vi "Script Work VIs.vi"(6 "Context":refnum<vi>, 7 "New Block Config":T1={"Name"="", "Actions"={"Init"=FALSE, "Start"=FALSE, "Run"=TRUE, "Stop"=FALSE, "Close"=FALSE}, "IO Control"=FALSE, "New Project?"=FALSE, "Project"=refnum}, 8 "error in (no error)":errorcluster, 11 "Worker Library Path":path) -> (0 "error out":errorcluster)   [LabVIEW 2022 SP3, in "FlexBlocks Support.lvlib"]
uses:
  FlexBlocks Support.lvlib
  <vilib>/Utility/traverseref.llb/TRef TravTarget.ctl
  Worker Action.ctl
  <vilib>/Utility/error.llb/Trim Whitespace One-Sided.vi
  <vilib>/Utility/traverseref.llb/VI Scripting - Traverse.lvlib
  Action Selections.ctl
  New Block Config.ctl
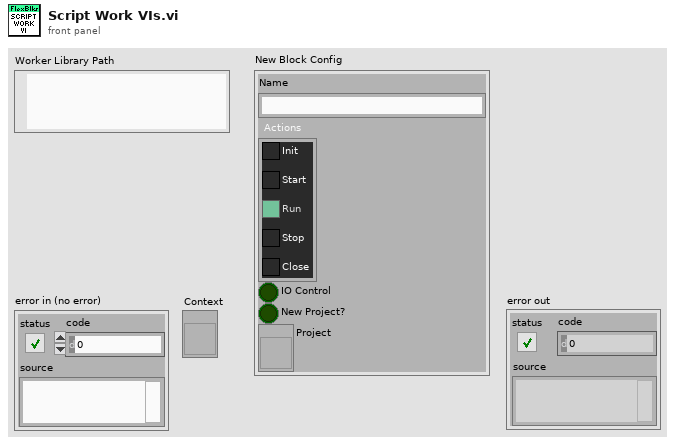
[diagram p1: front panel]
types:
  T1 = typedef "FlexBlocks Support.lvlib/New Block Config.ctl" = cluster{"Name":string, "Actions":T2, "IO Control":bool, "New Project?":bool, "Project":refnum<vi>}
  T2 = typedef "FlexBlocks Support.lvlib/Action Selections.ctl" = cluster{"Init":bool, "Start":bool, "Run":bool, "Stop":bool, "Close":bool}
  T3 = enum32{"invalid lock state", "Not Locked", "Locked (No Password)", "Password-protected"}
  T4 = typedef "TRef TravTarget.ctl" = enum16{"FP", "BD", "Other"}
  T5 = typedef "FlexBlocks Support.lvlib/Worker Action.ctl" = enum16{"Init", "Start", "Run", "Stop", "Close"}
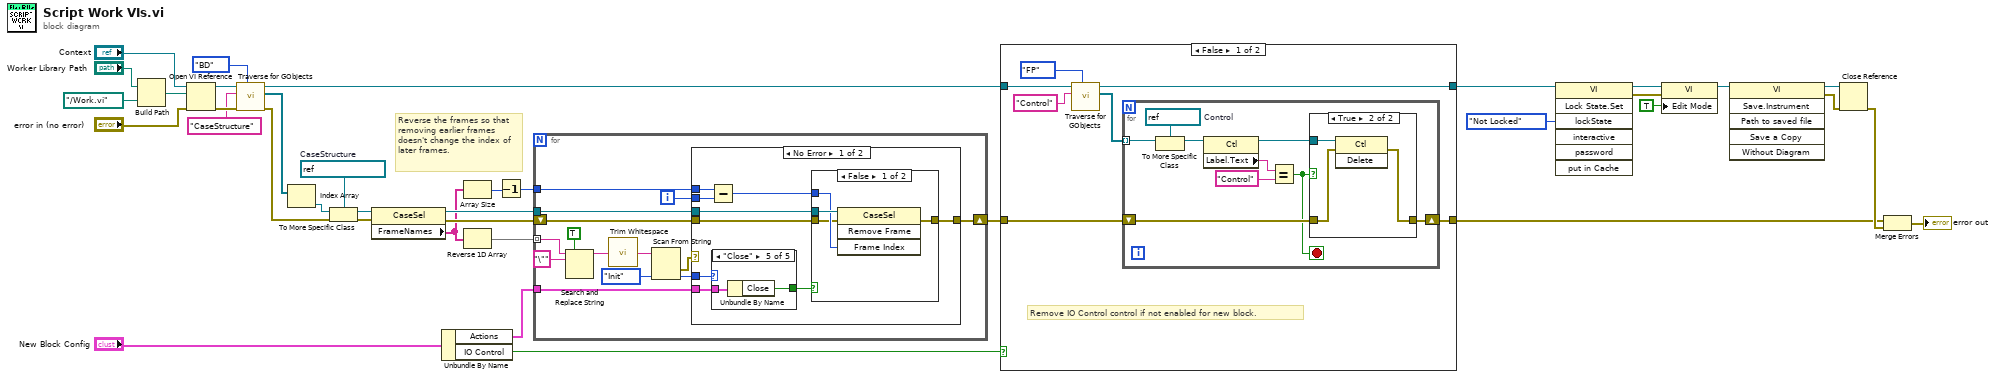
[diagram p0: block diagram]
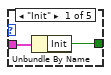
[diagram p5: hidden frame]
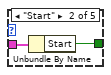
[diagram p6: hidden frame]
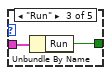
[diagram p7: hidden frame]
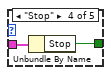
[diagram p8: hidden frame]
diagram:
  w27 = refnum<vi> refnum  # CaseStructure
  # "Reverse the frames so that removing earlier frames doesn't change the index of later frames."
  n1 = Build Path(base path="Worker Library Path", name or relative path=path "../Work.vi") -> (appended path=w35:path)
  n2 = Open VI Reference(application reference (local)="Context", vi path=w35, error in (no error)="error in (no error)") -> (vi reference=w33:refnum<vi>, error out=w31:errorcluster)  [unwired: 3 in]
  n3 = call <vilib>:"Traverse for GObjects.vi"("Traverse Target"=TRef_TravTarget."BD", "error in (no error)"=w31, "Class Name"="CaseStructure", "VI Refnum"=w33) -> ("error out"=w25:errorcluster, "References"=w29:refnum<vi>[], "dup VI Refnum"=w4:refnum<vi>)  [unwired: 4 in, 1 out]
  n4 = Index Array(array=w29) -> (element=w28:refnum<vi>)  [unwired: 1 in]
  n5 = To More Specific Class(target class=w27, reference=w28, error in=w25) -> (specific class reference=w26:refnum<vi>, error out=w24:errorcluster)
  n6 = property class="CaseSel"(reference=w26, error in=w24) -> (reference out=w23:refnum<vi>, error out=w22:errorcluster, "FrameNames"=w15:string[])
  n7 = Unbundle By Name("New Block Config") -> ("Actions"=w6:T2, "IO Control"=w5:bool)
  n8 = Array Size(array=w15) -> (size(s)=w14:i32)
  n9 = Reverse 1D Array(array=w15) -> (reversed array=w16:string[])
  n10 = Decrement(x=w14) -> (x-1=w13:i32)
  n11 = for {
    tunnel: w16 -> [w43] mode=indexing
    tunnel: w6 -> [w51]
    tunnel: w23 -> [w50]
    shift-right: [w44] -> w2
    shift-left: w22 -> [w45]
    tunnel: w13 -> [w38]
    i -> [w46]
    n12 = Search and Replace String(replace all?=TRUE ("replace all? (F)"), input string=w43, search string="\"") -> (result string=w42:string)  [unwired: 5 in, 3 out]
    n13 = call <vilib>:"Trim Whitespace.vi"("string"=w42) -> ("trimmed string"=w39:string)  [unwired: 1 in]
    n14 = Scan From String(input string=w39, default 1=Worker_Action."Init" ("Action")) -> (error out=w47:errorcluster, output 1=w48:T5)  [unwired: 3 in, 2 out]
    n15 = case shown="No Error" w47 {
      tunnel: w51 -> [w52 _]
      tunnel: w50 -> [w58 _]
      tunnel: w48 -> [w60 _]
      tunnel: w46 -> [w54 _]
      tunnel: w45 -> [w57 w76]
      tunnel: [w56 w76] -> w44
      tunnel: w38 -> [w55 _]
      frame No Error {
        n16 = Subtract(x=w55, y=w54) -> (x-y=w53:i32)
        n17 = case shown="\"Close\"" w60 {
          tunnel: w52 -> [w67 w69 w71 w73 w75]
          tunnel: [w66 w68 w70 w72 w74] -> w59
          frame "Init" {
            n18 = Unbundle By Name(w67) -> ("Init"=w66:bool)
          }
          frame "Start" {
            n19 = Unbundle By Name(w69) -> ("Start"=w68:bool)
          }
          frame "Run" {
            n20 = Unbundle By Name(w71) -> ("Run"=w70:bool)
          }
          frame "Stop" {
            n21 = Unbundle By Name(w73) -> ("Stop"=w72:bool)
          }
          frame "Close" {
            n22 = Unbundle By Name(w75) -> ("Close"=w74:bool)
          }
        }
        n23 = case shown="False" w59 {
          tunnel: w53 -> [w63 _]
          tunnel: w58 -> [w64 _]
          tunnel: w57 -> [w62 w65]
          tunnel: [w61 w65] -> w56
          frame False {
            n24 = invoke class="CaseSel" method="Remove Frame"(reference=w64, error in=w62, "Frame Index"=w63) -> (error out=w61:errorcluster)  [unwired: 1 in, 3 out]
          }
          frame True {
          }
        }
      }
      frame Error {
        # "Default Case, always stays"
      }
    }
  }
  n25 = case shown="False" w5 {
    tunnel: w4 -> [w83 w98]
    tunnel: [w79 w98] -> w3
    tunnel: w2 -> [w78 w97]
    tunnel: [w77 w97] -> w1
    frame False {
      # "Remove IO Control control if not enabled for new block."
      n26 = call <vilib>:"Traverse for GObjects.vi"("Traverse Target"=TRef_TravTarget."FP", "Class Name"="Control", "VI Refnum"=w83) -> ("References"=w80:refnum<vi>[], "dup VI Refnum"=w79:refnum<vi>)  [unwired: 5 in, 2 out]
      n27 = for {
        tunnel: w80 -> [w92] mode=indexing
        shift-right: [w86] -> w77
        shift-left: w78 -> [w87]
        stop <- w84 stop-if-true
        w91 = refnum<vi> refnum  # Control
        n28 = To More Specific Class(target class=w91, reference=w92) -> (specific class reference=w90:refnum<vi>)  [unwired: 1 in, 1 out]
        n29 = property class="Ctl"(reference=w90) -> (reference out=w85:refnum<vi>, "Label.Text"=w89:string)  [unwired: 1 in, 1 out]
        n30 = Equal?(x=w89, y="Control") -> (x = y?=w84:bool)
        n31 = case shown="True" w84 {
          tunnel: w85 -> [_ w96]
          tunnel: w87 -> [w93 w95]
          tunnel: [w93 w94] -> w86
          frame False {
          }
          frame True {
            n32 = invoke class="Ctl" method="Delete"(reference=w96, error in=w95) -> (error out=w94:errorcluster)  [unwired: 1 in, 2 out]
          }
        }
      }
    }
    frame True {
    }
  }
  n33 = invoke class="VI" method="Lock State.Set"(reference=w3, "lockState"=T3."Not Locked" ("Lock State")) -> (reference out=w9:refnum<vi>, error out=w8:errorcluster)  [unwired: 5 in, 5 out]
  n34 = property class="VI"(reference=w9, error in=w8, "Edit Mode"=TRUE ("Edit Mode On Open")) -> (reference out=w12:refnum<vi>)  [unwired: 1 out]
  n35 = invoke class="VI" method="Save.Instrument"(reference=w12) -> (reference out=w21:refnum<vi>, error out=w20:errorcluster)  [unwired: 5 in, 4 out]
  n36 = Close Reference(reference=w21, error in (no error)=w20) -> (error out=w19:errorcluster)
  n37 = Merge Errors(w1, w19) -> (→"error out":errorcluster)
